vi "TDMS.Open.Wait.vi"(8 "error in (no error)":errorcluster, 10 "operation (open read-only)":T1(ring)=enum."open (read-only)", 11 "file path":path) -> (0 "error out":errorcluster, 3 "tdms file out":refnum<k34>)   [LabVIEW 2016]
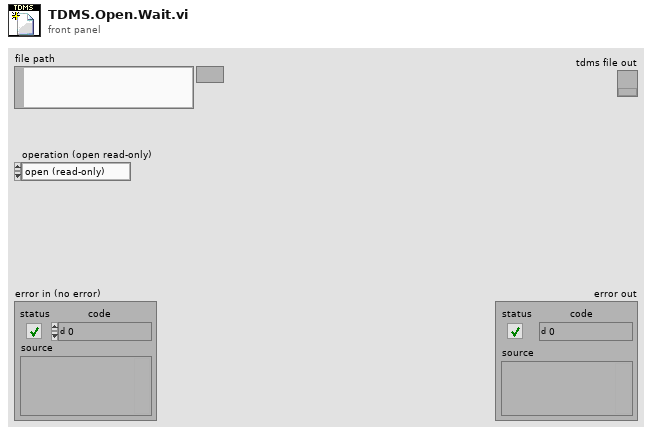
[diagram p1: front panel]
types:
  T1 = enum16{"open", "open or create", "create or replace", "create", "open (read-only)"}
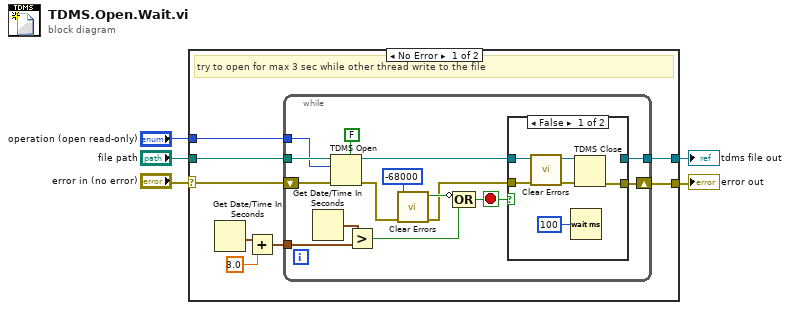
[diagram p0: block diagram]
diagram:
  n1 = case shown="No Error" "error in (no error)" {
    selector: "error in (no error)" -> [w12 w36]
    tunnel: "file path" -> [w13 _]
    tunnel: [w11 _] -> w3
    tunnel: [w7 w36] -> w2
    tunnel: "operation (open read-only)" -> [w6 _]
    frame No Error {
      # "try to open for max 3 sec while other thread write to the file"
      n2 = Get Date/Time In Seconds() -> (seconds since 1Jan1904=w9:timestamp)
      n3 = Add(x=w9, y=3.0) -> (x+y=w8:timestamp)
      n4 = while {
        tunnel: w13 -> [w28]
        tunnel: [w24] -> w11
        tunnel: w8 -> [w21]
        tunnel: w6 -> [w18]
        shift-right: [w16] -> w7
        shift-left: w12 -> [w27]
        stop <- w20 stop-if-true
        n5 = Get Date/Time In Seconds() -> (seconds since 1Jan1904=w22:timestamp)
        n6 = TDMS Open(5:FALSE ("create index file? (T)"), 8:w27, 10:w18, 11:w28) -> (0:w17:errorcluster, 3:w25:refnum<k34>)  [unwired: 3 in]
        n7 = Greater?(x=w22, y=w21) -> (0:w19:bool)
        n8 = call <vilib>:"Clear Errors.vi"("error in (no error)"=w17, "specific error code to clear (0: all)"=-68000) -> ("error out"=w15:errorcluster, "specific error cleared?"=w23:bool)  [unwired: 4 in]
        n9 = Compound Arithmetic op=OR(invert w23, w19) -> (w20:bool)
        n10 = case shown="False" w20 {
          tunnel: w25 -> [w33 w35]
          tunnel: [_ w35] -> w24
          tunnel: [w32 w34] -> w16
          tunnel: w15 -> [w31 w34]
          frame False {
            n11 = call <vilib>:"Clear Errors.vi"("error in (no error)"=w31) -> ("error out"=w30:errorcluster)  [unwired: 5 in, 1 out]
            n12 = Wait (ms)(milliseconds to wait=u32 100) -> ()  [unwired: 1 out]
            n13 = TDMS Close(8:w30, 11:w33) -> (0:w32:errorcluster)  [unwired: 1 out]
          }
          frame True {
          }
        }
      }
    }
    frame Error {
    }
  }
  "error out" <- w2
  "tdms file out" <- w3
